vi "HEWH Write Stats.vi"(4 "Debug All Stats":string[][](array[string])=[["Voltage (Volts) - Mean", "Voltage (Volts) - Standard Deviation", "Voltage (Volts) - Variance", "Voltage (Volts) - Max", "Voltage (Volts) - Min", "Current (Amps) - Mean", "Current (Amps) - Standard Deviation", "Current (Amps) - Variance", "Current (Amps) - Max", "Current (Amps) - Min", "Power (Watts) - Mean", "Power (Watts) - Standard Deviation", "Power (Watts) - Variance", "Power (Watts) - Max", "Power (Watts) - Min", "WattHours - Max", "WattHours - Min", "TC Tree (AVG) - Mean", "TC Tree (AVG) - Standard Deviation", "TC Tree (AVG) - Variance", "TC Tree (AVG) - Max", "TC Tree (AVG) - Min", "Flow Rate (GPM) - Mean", "Flow Rate (GPM) - Standard Deviation", "Flow Rate (GPM) - Variance", "Flow Rate (GPM) - Max", "Flow Rate (GPM) - Min", "Gallons (Gal) - Max", "Gallons (Gal) - Min", "RTD Out (°F) - Mean", "RTD Out (°F) - Standard Deviation", "RTD Out (°F) - Variance", "RTD Out (°F) - Max", "RTD Out (°F) - Min", "RTD In (°F) - Mean", "RTD In (°F) - Standard Deviation", "RTD In (°F) - Variance", "RTD In (°F) - Max", "RTD In (°F) - Min", "RTD Ambinet (°F) - Mean", "RTD Ambient (°F) - Standard Deviation", "RTD Ambinent (°F) - Variance", "RTD Ambinent (°F) - Max", "RTD Ambinent (°F) - Min", "TC Down (°F) - Mean", "TC Down (°F) - Standard Deviation", "TC Down (°F) - Variance", "TC Down (°F) - Max", "TC Down (°F) - Min", "TC1 (°F) - Mean", "TC1 (°F) - Standard Deviation", "TC1 (°F) - Variance", "TC1 (°F) - Max", "TC1 (°F) - Min", "TC2 (°F) - Mean", "TC2 (°F) - Standard Deviation", "TC2 (°F) - Variance", "TC2 (°F) - Max", "TC2 (°F) - Min", "TC3 (°F) - Mean", "TC3 (°F) - Standard Deviation", "TC3 (°F) - Variance", "TC3 (°F) - Max", "TC3 (°F) - Min", "TC4 (°F) - Mean", "TC4 (°F) - Standard Deviation", "TC4 (°F) - Variance", "TC4 (°F) - Max", "TC4 (°F) - Min", "TC5 (°F) - Mean", "TC5 (°F) - Standard Deviation", "TC5 (°F) - Variance", "TC5 (°F) - Max", "TC5 (°F) - Min", "TC6 (°F) - Mean", "TC6 (°F) - Standard Deviation", "TC6 (°F) - Variance", "TC6 (°F) - Max", "TC6 (°F) - Min", "Total Harmonic Distortion (%V) - Max", "Total Harmonic Distortion (%V) - Min", "Frequency (Hz) - Mean ", "Frequency (Hz) - Standard Deviation", "Frequency (Hz) - Variance", "Frequency (Hz) - Max", "Frequency (Hz) - Min", "Apparent Power (VA) - Mean", "Apparent Power (VA) - Standard Deviation", "Apparent Power (VA) - Variance", "Apparent Power (VA) - Max", "Apparent Power (VA) - Min", "Power Factor - Max", "Power Factor - Min", "Current Crest Factor - Max", "Current Crest Factor - Min", "Voltage Crest Factor - Max", "Voltage Crest Factor - Min", "Elapsed Time (Sec) - Max", "Elapsed Time (Sec) - Min", "Condition Value #1", "Draw Count"], ["1.000", "NaN", "NaN", "1.000", "1.000", "2.000", "NaN", "NaN", "2.000", "2.000", "3.000", "NaN", "NaN", "3.000", "3.000", "4.000", "4.000", "5.000", "NaN", "NaN", "5.000", "5.000", "6.000", "NaN", "NaN", "6.000", "6.000", "7.000", "7.000", "8.000", "NaN", "NaN", "8.000", "8.000", "9.000", "NaN", "NaN", "9.000", "9.000", "10.000", "NaN", "NaN", "10.000", "10.000", "11.000", "NaN", "NaN", "11.000", "11.000", "14.000", "NaN", "NaN", "14.000", "14.000", "15.000", "NaN", "NaN", "15.000", "15.000", "16.000", "NaN", "NaN", "16.000", "16.000", "17.000", "NaN", "NaN", "17.000", "17.000", "18.000", "NaN", "NaN", "18.000", "18.000", "19.000", "NaN", "NaN", "19.000", "19.000", "20.000", "20.000", "21.000", "NaN", "NaN", "21.000", "21.000", "22.000", "NaN", "NaN", "22.000", "22.000", "23.000", "23.000", "24.000", "24.000", "25.000", "25.000", "28.000", "28.000", "0.000", "27"]], 6 "Debug Mean SD Var Max Min Array":string[][](array[string])=[["Voltage (Volts) - Mean", "1.000"], ["Voltage (Volts) - Standard Deviation", "NaN"], ["Voltage (Volts) - Variance", "NaN"], ["Voltage (Volts) - Max", "1.000"], ["Voltage (Volts) - Min", "1.000"], ["Current (Amps) - Mean", "2.000"], ["Current (Amps) - Standard Deviation", "NaN"], ["Current (Amps) - Variance", "NaN"], ["Current (Amps) - Max", "2.000"], ["Current (Amps) - Min", "2.000"], ["Power (Watts) - Mean", "3.000"], ["Power (Watts) - Standard Deviation", "NaN"], ["Power (Watts) - Variance", "NaN"], ["Power (Watts) - Max", "3.000"], ["Power (Watts) - Min", "3.000"], ["WattHours - Max", "4.000"], ["WattHours - Min", "4.000"], ["TC Tree (AVG) - Mean", "5.000"], ["TC Tree (AVG) - Standard Deviation", "NaN"], ["TC Tree (AVG) - Variance", "NaN"], ["TC Tree (AVG) - Max", "5.000"], ["TC Tree (AVG) - Min", "5.000"], ["Flow Rate (GPM) - Mean", "6.000"], ["Flow Rate (GPM) - Standard Deviation", "NaN"], ["Flow Rate (GPM) - Variance", "NaN"], ["Flow Rate (GPM) - Max", "6.000"], ["Flow Rate (GPM) - Min", "6.000"], ["Gallons (Gal) - Max", "7.000"], ["Gallons (Gal) - Min", "7.000"], ["RTD Out (°F) - Mean", "8.000"], ["RTD Out (°F) - Standard Deviation", "NaN"], ["RTD Out (°F) - Variance", "NaN"], ["RTD Out (°F) - Max", "8.000"], ["RTD Out (°F) - Min", "8.000"], ["RTD In (°F) - Mean", "9.000"], ["RTD In (°F) - Standard Deviation", "NaN"], ["RTD In (°F) - Variance", "NaN"], ["RTD In (°F) - Max", "9.000"], ["RTD In (°F) - Min", "9.000"], ["RTD Ambinet (°F) - Mean", "10.000"], ["RTD Ambient (°F) - Standard Deviation", "NaN"], ["RTD Ambinent (°F) - Variance", "NaN"], ["RTD Ambinent (°F) - Max", "10.000"], ["RTD Ambinent (°F) - Min", "10.000"], ["TC Down (°F) - Mean", "11.000"], ["TC Down (°F) - Standard Deviation", "NaN"], ["TC Down (°F) - Variance", "NaN"], ["TC Down (°F) - Max", "11.000"], ["TC Down (°F) - Min", "11.000"], ["TC1 (°F) - Mean", "14.000"], ["TC1 (°F) - Standard Deviation", "NaN"], ["TC1 (°F) - Variance", "NaN"], ["TC1 (°F) - Max", "14.000"], ["TC1 (°F) - Min", "14.000"], ["TC2 (°F) - Mean", "15.000"], ["TC2 (°F) - Standard Deviation", "NaN"], ["TC2 (°F) - Variance", "NaN"], ["TC2 (°F) - Max", "15.000"], ["TC2 (°F) - Min", "15.000"], ["TC3 (°F) - Mean", "16.000"], ["TC3 (°F) - Standard Deviation", "NaN"], ["TC3 (°F) - Variance", "NaN"], ["TC3 (°F) - Max", "16.000"], ["TC3 (°F) - Min", "16.000"], ["TC4 (°F) - Mean", "17.000"], ["TC4 (°F) - Standard Deviation", "NaN"], ["TC4 (°F) - Variance", "NaN"], ["TC4 (°F) - Max", "17.000"], ["TC4 (°F) - Min", "17.000"], ["TC5 (°F) - Mean", "18.000"], ["TC5 (°F) - Standard Deviation", "NaN"], ["TC5 (°F) - Variance", "NaN"], ["TC5 (°F) - Max", "18.000"], ["TC5 (°F) - Min", "18.000"], ["TC6 (°F) - Mean", "19.000"], ["TC6 (°F) - Standard Deviation", "NaN"], ["TC6 (°F) - Variance", "NaN"], ["TC6 (°F) - Max", "19.000"], ["TC6 (°F) - Min", "19.000"], ["Total Harmonic Distortion (%V) - Max", "20.000"], ["Total Harmonic Distortion (%V) - Min", "20.000"], ["Frequency (Hz) - Mean ", "21.000"], ["Frequency (Hz) - Standard Deviation", "NaN"], ["Frequency (Hz) - Variance", "NaN"], ["Frequency (Hz) - Max", "21.000"], ["Frequency (Hz) - Min", "21.000"], ["Apparent Power (VA) - Mean", "22.000"], ["Apparent Power (VA) - Standard Deviation", "NaN"], ["Apparent Power (VA) - Variance", "NaN"], ["Apparent Power (VA) - Max", "22.000"], ["Apparent Power (VA) - Min", "22.000"], ["Power Factor - Max", "23.000"], ["Power Factor - Min", "23.000"], ["Current Crest Factor - Max", "24.000"], ["Current Crest Factor - Min", "24.000"], ["Voltage Crest Factor - Max", "25.000"], ["Voltage Crest Factor - Min", "25.000"], ["Elapsed Time (Sec) - Max", "28.000"], ["Elapsed Time (Sec) - Min", "28.000"], ["Condition Value #1", "0.000"], ["Draw Count", "27"]], 8 "Error In":errorcluster, 10 "Mean SD Var Max Min Array":string[][](array[string]), 11 "All Draw Stats In":string[][](array[string])) -> (0 "Error Out":errorcluster, 3 "All Draw Stats Out":string[][](array[string]))   [LabVIEW 2019]
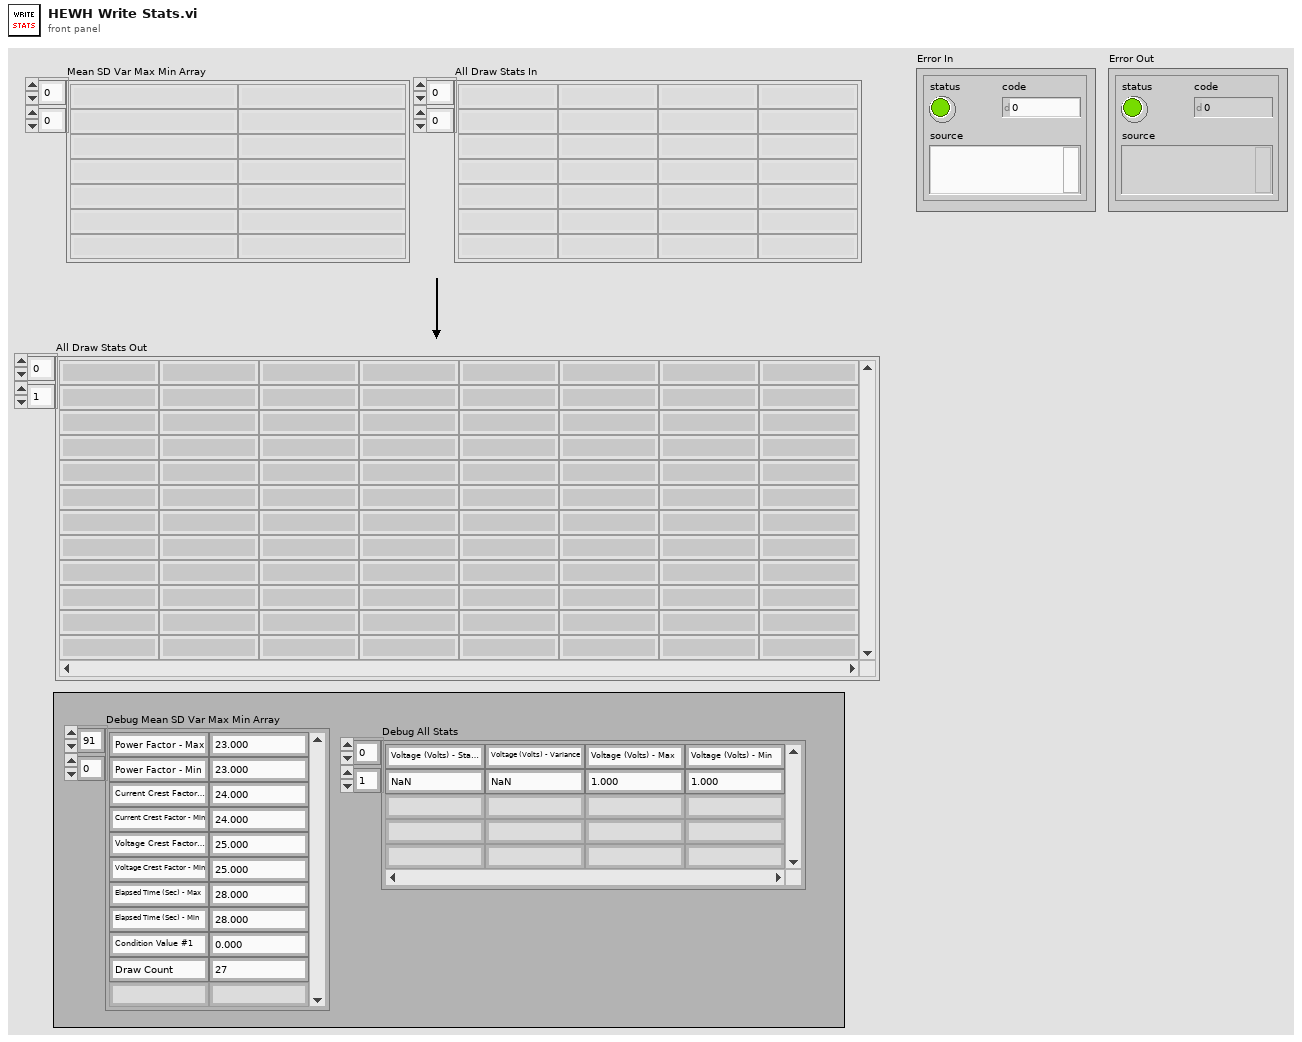
[diagram p1: front panel]
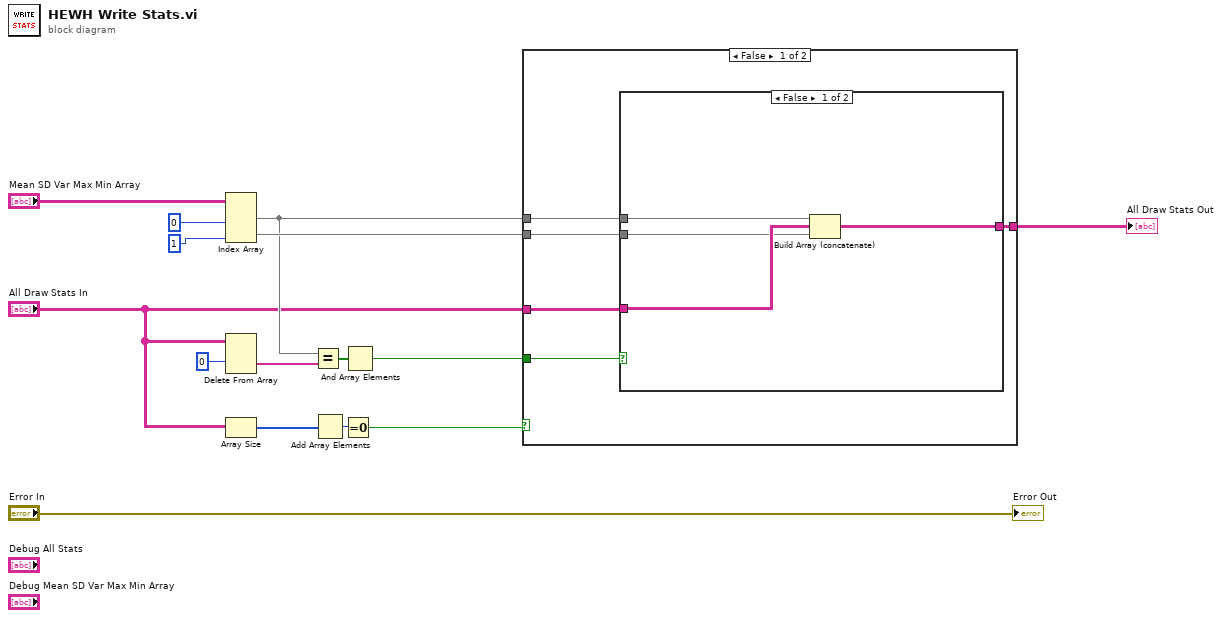
[diagram p0: block diagram]
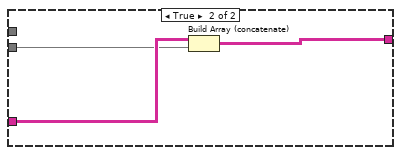
[diagram p2: hidden frame]
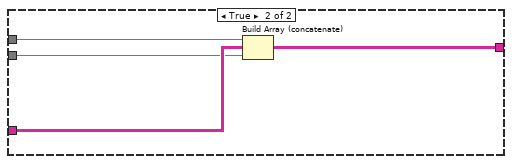
[diagram p3: hidden frame]
diagram:
  n1 = Index Array(array="Mean SD Var Max Min Array", index (col) #1=0 ("disabled index (col)"), index (col) #2=1 ("disabled index (col)")) -> (element #1=w8:string[], element #2=w15:string[])  [unwired: 2 in]
  n2 = Delete From Array(array="All Draw Stats In", index (row)=0) -> (deleted portion=w9:string[])  [unwired: 2 in, 1 out]
  n3 = Array Size(array="All Draw Stats In") -> (size(s)=w6:i32[])
  n4 = Equal?(x=w8, y=w9) -> (x = y?=w7:bool[])
  n5 = Add Array Elements(numeric array=w6) -> (sum=w5:i32)
  n6 = Equal To 0?(x=w5) -> (x = 0?=w3:bool)
  n7 = And Array Elements(Boolean array=w7) -> (logical AND=w4:bool)
  n8 = case shown="False" w3 {
    tunnel: w15 -> [w20 w28]
    tunnel: [w19 w30] -> w12
    tunnel: w8 -> [w18 w31]
    tunnel: "All Draw Stats In" -> [w17 w29]
    tunnel: w4 -> [w16 _]
    frame False {
      n9 = case shown="False" w16 {
        tunnel: w17 -> [w24 w27]
        tunnel: w20 -> [w23 w26]
        tunnel: [w22 w25] -> w19
        tunnel: w18 -> [w21 _]
        frame False {
          n10 = Build Array (concatenate)(w21, w24, w23) -> (w22:string[][])
        }
        frame True {
          n11 = Build Array (concatenate)(w27, w26) -> (w25:string[][])
        }
      }
    }
    frame True {
      n12 = Build Array (concatenate)(w31, w29, w28) -> (w30:string[][])
    }
  }
  "All Draw Stats Out" <- w12
  "Error Out" <- "Error In"
